vi "Station_1_Detection.vi"() -> ()   [LabVIEW 2011]
uses:
  <vilib>/userDefined/High Color/IMAQdx.ctl
  <vilib>/Utility/file.llb/Write To Spreadsheet File (string).vi
  <vilib>/vision/driver/NI_Vision_Acquisition_Software.lvlib
  <vilib>/vision/NI_Vision_Development_Module.lvlib
panel:
  in  "Minimum Match Score":sgl=900.0
  in  "Text File Information":path=path "C:/Users/Kevin/Documents/Masters (Semester 2)/MEng Thesis/LabVIEW_CompleteV3/TextFiles"
  in  "Saved Image Location":path=path "C:/Users/Kevin/Documents/Masters (Semester 2)/MEng Thesis/LabVIEW_CompleteV3/ImagesFiles"
  in  "Template Location":path=path "C:/Users/Kevin/Documents/Masters (Semester 2)/MEng Thesis/LabVIEW_CompleteV3/Templates/Shape"
  in  "Colour Selection":enum32{"Default", "Automatic", "Manual"}(radio)
  out "Created Colours":u32[](array[colorbox])
  out "Switch Ready":bool
  out "Colours Ready":bool
  in  "Run Search":bool
  out "Running":bool
  out "Results Cluster":T2 {"Colour Code" format="%.0x"}
  out "Image File":string
  in  "Selected Colours":u32[](array[colorbox])
  in  "Full Program Stop":bool
  out "Image Out":T1(plugin-control)
  out "Results Information":string[][](table)
  out "No Shapes Found":bool
  out "Shape(s) Found":bool
  out "Image Iteration":u32
  out "Saving":bool
  out "Image Name":string
  # "Kevin Mulkearn\n11124725\nUniversity of Limerick"
  # "Instructions:\n1. Select File Locations.\n2. Run application.\n3. Generate/Select Colours.\n4. Select 'START' button."
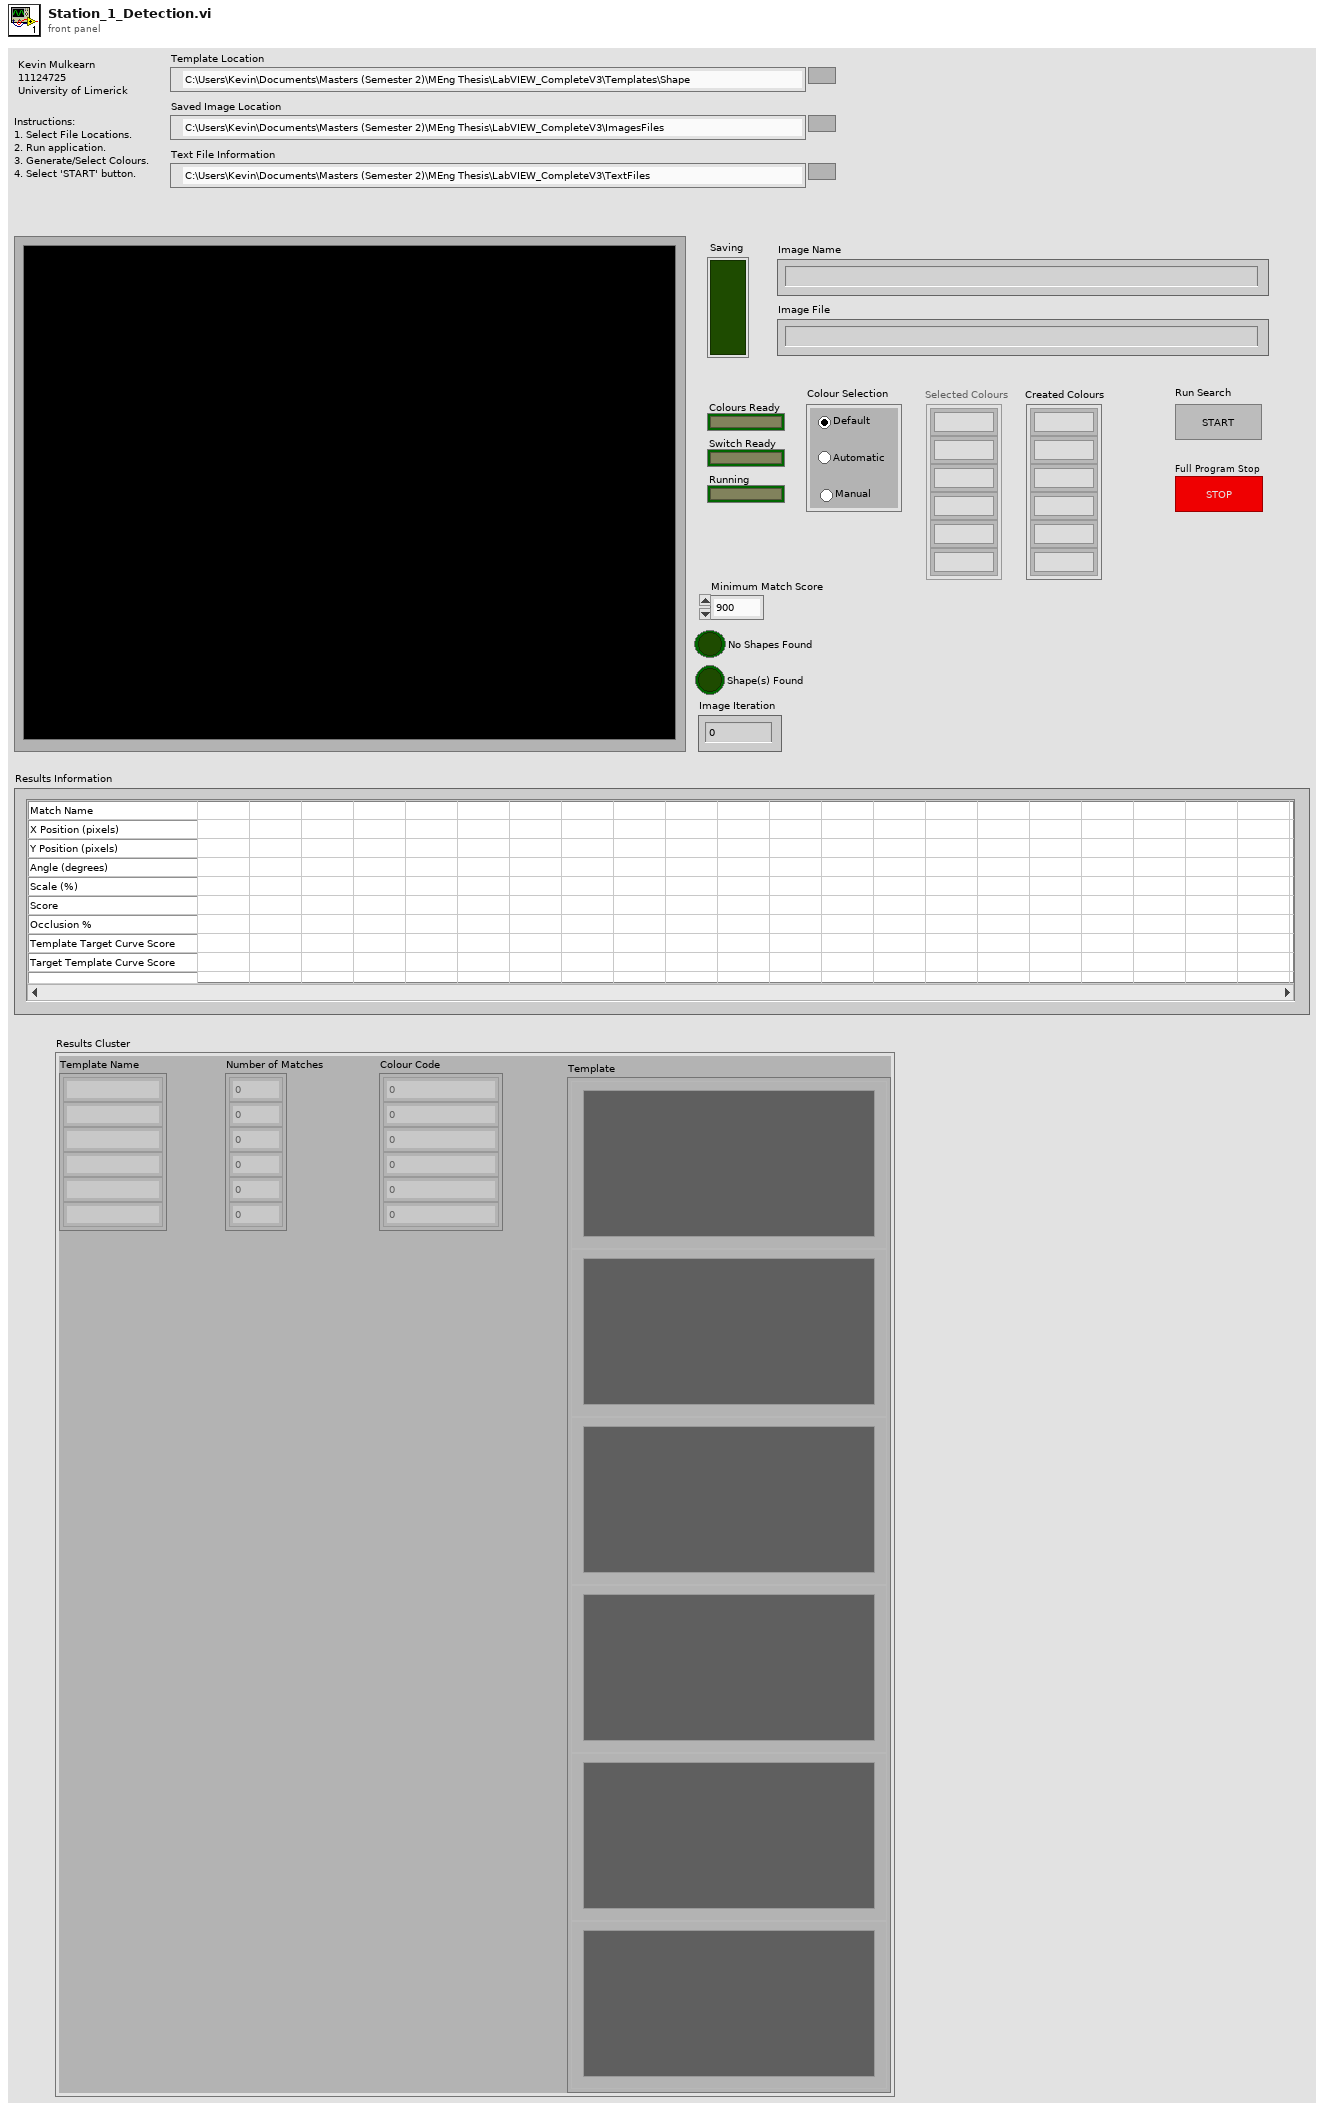
[diagram p1: front panel]
types:
  T1 = typedef "IMAQ Image.ctl" = refnum<image>
  T2 = cluster{"Number of Matches":i32[], "Colour Code":u32[], "Template":T1[], "Template Name":string[]}
  T3 = typedef "IMAQdx.ctl" = refnum<k21>
  T4 = cluster{"Rotation":bool, "Scale":bool, "Occlusion":bool, "Reserved":bool, "Reserved":bool, "Reserved":bool}
  T5 = cluster{"Match Geometric Pattern Setup Data":string, "Number of Matches":i32, "Minimum Match Score":sgl}
  T6 = typedef "IMAQ GM Multiple Template.ctl" = refnum<k20>
  T7 = enum8{"Enabled", "Disabled", "Disabled and Grayed Out"}
  T8 = typedef "IMAQ GM Match Report.ctl" = cluster{"Position":cluster{"x":sgl, "y":sgl}, "Angle":sgl, "Scale":sgl, "Score":sgl, "Bounding Box":cluster{"x":sgl, "y":sgl}[], "Contrast Reversed":bool, "Occlusion %":sgl, "Template Target Curve Score":sgl, "Target Template Curve Score":sgl, "Correlation Score":sgl}
  T9 = cluster{"Number of Matches":i32[], u32[], T1[], string[]}
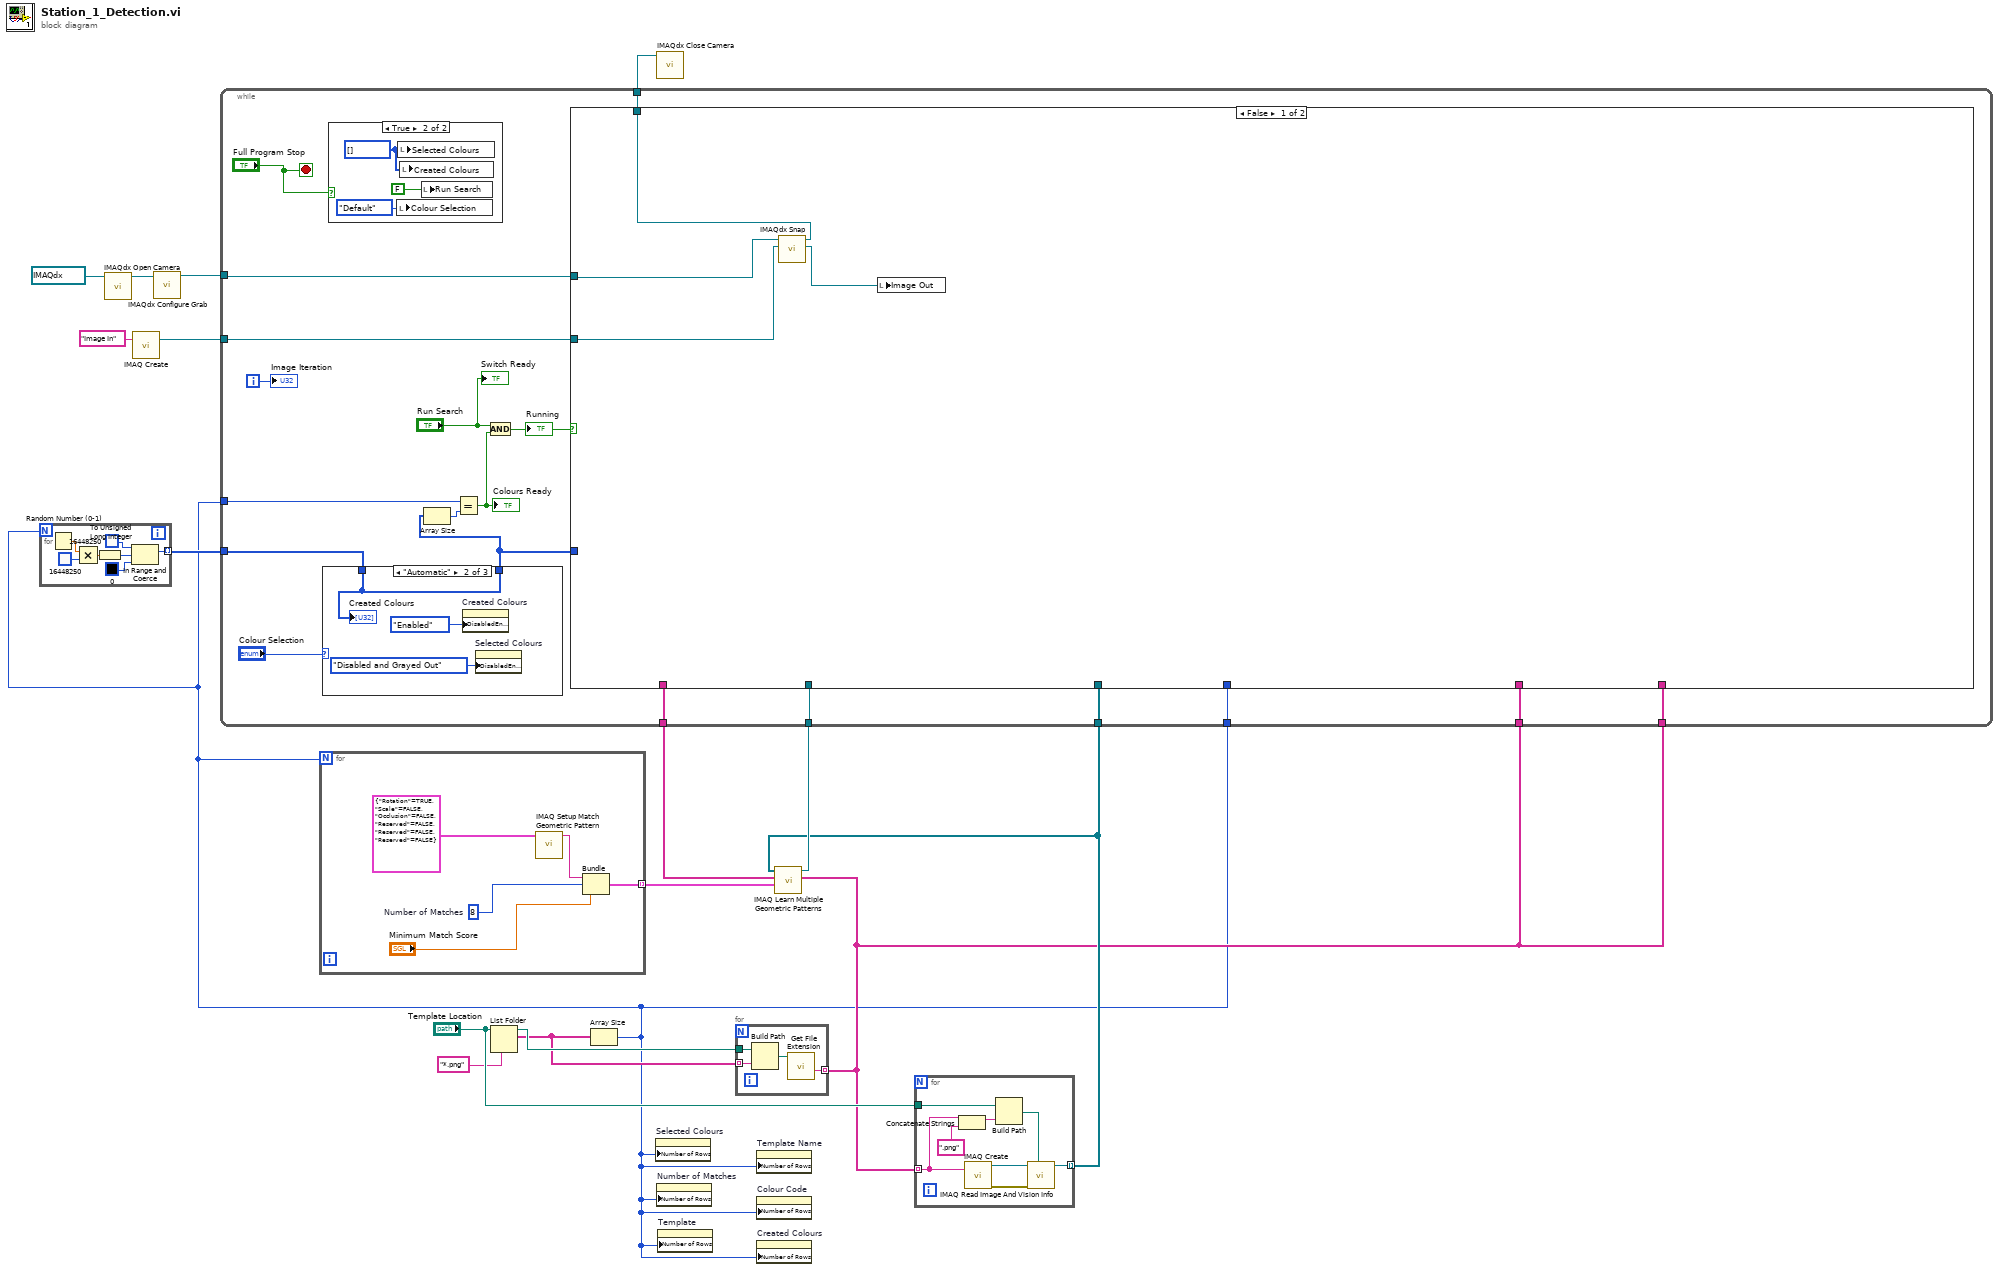
[diagram p0: block diagram]
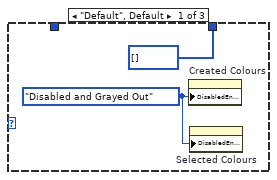
[diagram p2: hidden frame]
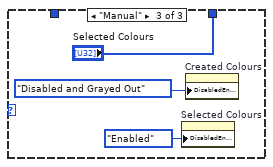
[diagram p3: hidden frame]
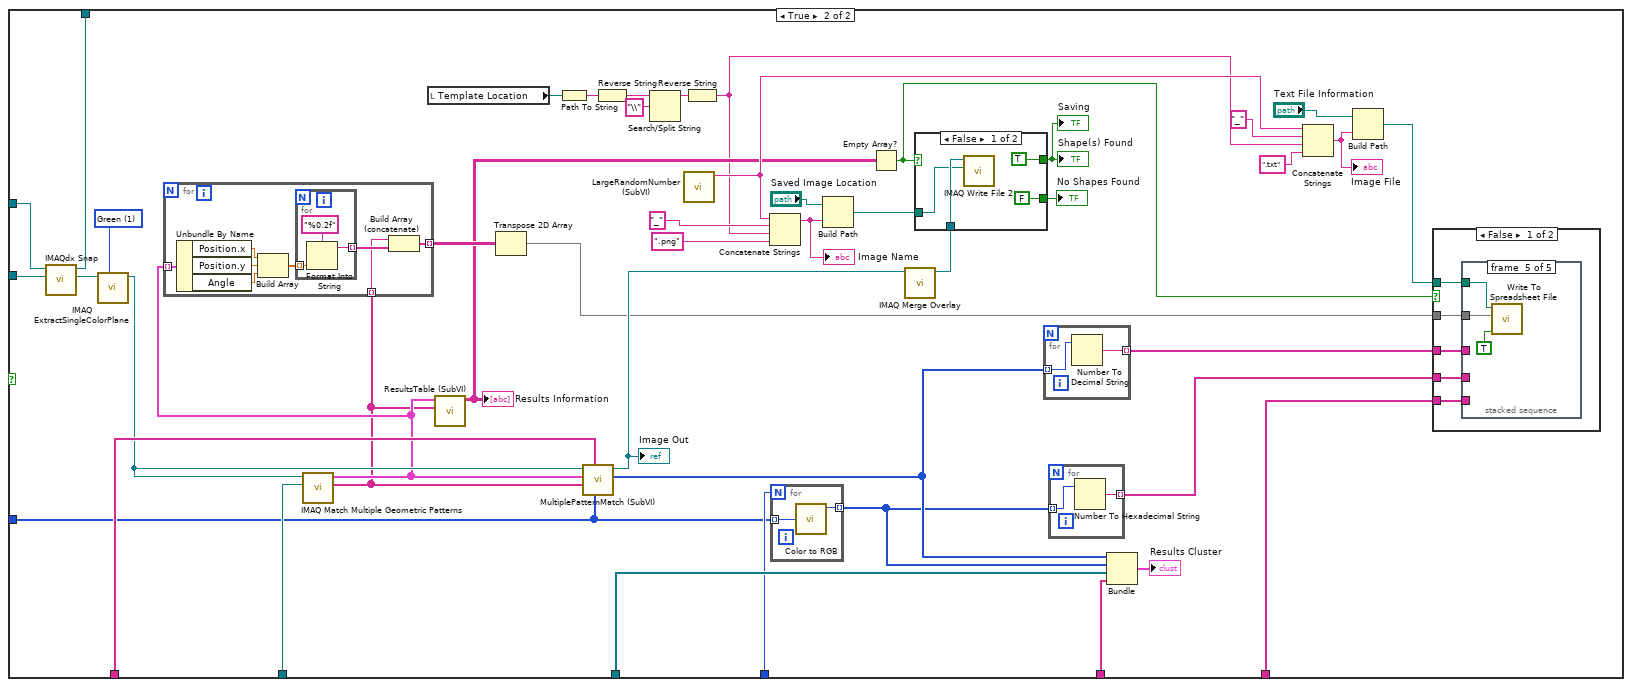
[diagram p5: hidden frame]
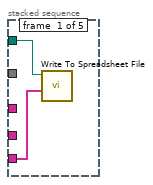
[diagram p6: hidden frame]
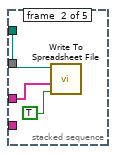
[diagram p7: hidden frame]
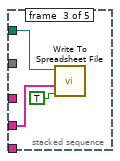
[diagram p8: hidden frame]
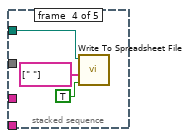
[diagram p9: hidden frame]
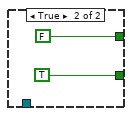
[diagram p11: hidden frame]
diagram:
  n1 = call <vilib>:"IMAQdx Open Camera.vi"("Session In"=T3 "cam2") -> ("Session Out"=w15:T3)  [unwired: 9 in, 1 out]
  n2 = call "IMAQ Create"("Image Name"="Image In") -> ("New Image"=w11:T1)  [unwired: 4 in, 1 out]
  n3 = call <vilib>:"IMAQdx Configure Grab.vi"("Session In"=w15) -> ("Session Out"=w14:T3)  [unwired: 9 in, 1 out]
  n4 = List Folder(path="Template Location", pattern="*.png") -> (path out=w6:path, filenames=w5:string[])  [unwired: 2 in, 2 out]
  n5 = Array Size(array=w5) -> (size(s)=w1:i32)
  n6 = for {
    N: w1 -> [_]
    tunnel: [w17] -> w2 mode=indexing
    n7 = Random Number (0-1)() -> (number: 0 to 1=w18:dbl)
    n8 = Multiply(x=w18, y=u32 16448250 ("Lightest Limit 2")) -> (x*y=w22:dbl)
    n9 = To Unsigned Long Integer(number=w22) -> (unsigned 32bit integer=w23:u32)
    n10 = In Range and Coerce(upper limit=u32 16448250 ("Lightest Limit"), x=w23, lower limit=u32 0 ("Darkest Limit")) -> (coerced(x)=w17:u32)  [unwired: 1 out]
  }
  n11 = for {
    N: w1 -> [_]
    tunnel: [w26] -> w10 mode=indexing
    w25 = 8  # Number of Matches
    n12 = call "IMAQ Setup Match Geometric Pattern"("Match Mode"=T4 {"Rotation"=TRUE, "Scale"=FALSE, "Occlusion"=FALSE, "Reserved"=FALSE, "Reserved"=FALSE, "Reserved"=FALSE}) -> ("Match Geometric Pattern Setup Data"=w27:string)  [unwired: 9 in, 1 out]
    n13 = Bundle("Match Geometric Pattern Setup Data"=w27, "Number of Matches"=w25, "Minimum Match Score"="Minimum Match Score") -> (w26:T5)  [unwired: 1 in]
  }
  n14 = property on="Selected Colours" class="Arr (strict)"("Number of Rows"=w1) -> ()  [unwired: 2 in, 2 out]
  n15 = property on="Number of Matches" class="Arr (strict)"("Number of Rows"=w1) -> ()  [unwired: 2 in, 2 out]
  n16 = property on="Template" class="Arr (strict)"("Number of Rows"=w1) -> ()  [unwired: 2 in, 2 out]
  n17 = for {
    tunnel: w6 -> [w32]
    tunnel: w5 -> [w31] mode=indexing
    tunnel: [w29] -> w3 mode=indexing
    n18 = Build Path(base path=w32, name or relative path=w31) -> (appended path=w30:path)
    n19 = call <vilib>:"Get File Extension.vi"("file"=w30) -> ("filename without extension"=w29:string)  [unwired: 7 in, 3 out]
  }
  n20 = property on="Template Name" class="Arr (strict)"("Number of Rows"=w1) -> ()  [unwired: 2 in, 2 out]
  n21 = property on="Colour Code" class="Arr (strict)"("Number of Rows"=w1) -> ()  [unwired: 2 in, 2 out]
  n22 = property on="Created Colours" class="Arr (strict)"("Number of Rows"=w1) -> ()  [unwired: 2 in, 2 out]
  n23 = for {
    tunnel: w3 -> [w38] mode=indexing
    tunnel: [w39] -> w7 mode=indexing
    tunnel: "Template Location" -> [w34]
    n24 = Concatenate Strings(w38, ".png" ("string")) -> (w37:string)
    n25 = call "IMAQ Create"("Image Name"=w38) -> ("New Image"=w40:T1, "error out"=w35:errorcluster)  [unwired: 3 in, 1 out]
    n26 = Build Path(base path=w34, name or relative path=w37) -> (appended path=w33:path)
    n27 = call "IMAQ Read Image And Vision Info"("File Path"=w33, "error in (no error)"=w35, "Image"=w40) -> ("Image Out"=w39:T1)  [unwired: 1 in, 7 out]
  }
  n28 = call "IMAQ Learn Multiple Geometric Patterns"("Default Match Options"=w10, "Template Labels"=w3, "Template Images"=w7) -> ("Multiple Template (out)"=w9:T6)  [unwired: 7 in, 1 out]
  n29 = while {
    tunnel: w14 -> [w59]
    tunnel: [w57] -> w13
    tunnel: w11 -> [w58]
    tunnel: w9 -> [w56]
    tunnel: w3 -> [w54]
    tunnel: w7 -> [w53]
    tunnel: w3 -> [w51]
    tunnel: w3 -> [w52]
    tunnel: w1 -> [w50]
    tunnel: w1 -> [w45]
    tunnel: w2 -> [w42]
    i -> [w55]
    stop <- "Full Program Stop" stop-if-true
    n30 = case shown="\"Automatic\"" "Colour Selection" {
      tunnel: [u32[] [] ("Select Colours") w64 "Selected Colours"] -> w43
      tunnel: w42 -> [_ w64 _]
      frame "Default", Default {
        w60 = T7."Disabled and Grayed Out" ("Disabled")
        n31 = property on="Created Colours" class="Arr (strict)"("DisabledEnum"=w60) -> ()  [unwired: 2 in, 2 out]
        n32 = property on="Selected Colours" class="Arr (strict)"("DisabledEnum"=w60) -> ()  [unwired: 2 in, 2 out]
      }
      frame "Automatic" {
        n33 = property on="Created Colours" class="Arr (strict)"("DisabledEnum"=T7."Enabled" ("Disabled")) -> ()  [unwired: 2 in, 2 out]
        n34 = property on="Selected Colours" class="Arr (strict)"("DisabledEnum"=T7."Disabled and Grayed Out" ("Disabled")) -> ()  [unwired: 2 in, 2 out]
        "Created Colours" <- w64
      }
      frame "Manual" {
        n35 = property on="Selected Colours" class="Arr (strict)"("DisabledEnum"=T7."Enabled" ("Disabled")) -> ()  [unwired: 2 in, 2 out]
        n36 = property on="Created Colours" class="Arr (strict)"("DisabledEnum"=T7."Disabled and Grayed Out" ("Disabled")) -> ()  [unwired: 2 in, 2 out]
      }
    }
    n37 = case shown="True" "Full Program Stop" {
      frame False {
      }
      frame True {
        w68 = u32[] []
        n38 = local write "Colour Selection"(enum32{"Default", "Automatic", "Manual"}."Default" ("Colour Selection Method")) -> ()
        n39 = local write "Selected Colours"(w68) -> ()
        n40 = local write "Created Colours"(w68) -> ()
        n41 = local write "Run Search"(FALSE ("Boolean")) -> ()
      }
    }
    n42 = Array Size(array=w43) -> (size(s)=w46:i32)
    n43 = Equal?(x=w45, y=w46) -> (x = y?=w47:bool)
    "Colours Ready" <- w47
    n44 = And(x="Run Search", y=w47) -> (x .and. y?=w49:bool)
    "Running" <- w49
    n45 = case shown="False" w49 {
      tunnel: w59 -> [w74 w119]
      tunnel: w58 -> [w73 w118]
      tunnel: [w71 w117] -> w57
      tunnel: w56 -> [_ w114]
      tunnel: w54 -> [_ w107]
      tunnel: w53 -> [_ w104]
      tunnel: w52 -> [_ w94]
      tunnel: w51 -> [_ w87]
      tunnel: w50 -> [_ w86]
      tunnel: w43 -> [_ w85]
      frame False {
        n46 = call <vilib>:"IMAQdx Snap.vi"("Image In"=w73, "Session In"=w74) -> ("Image Out"=w72:T1, "Session Out"=w71:T3)  [unwired: 7 in, 1 out]
        n47 = local write "Image Out"(w72) -> ()
      }
      frame True {
        w116 = 1 items=["Red", "Green", "Blue", "Hue", "Saturation", "Luminance", "Value", "Intensity"] ("Color Plane")
        n48 = call <vilib>:"IMAQdx Snap.vi"("Image In"=w118, "Session In"=w119) -> ("Image Out"=w115:T1, "Session Out"=w117:T3)  [unwired: 7 in, 1 out]
        n49 = call "IMAQ ExtractSingleColorPlane"("Color Plane"=w116, "Image Src"=w115) -> ("Image Dst Out"=w105:T1)  [unwired: 8 in, 1 out]
        n50 = call "IMAQ Match Multiple Geometric Patterns"("Multiple Template"=w114, "Image"=w105) -> ("Matched Labels"=w84:string[], "Matches (pixel)"=w92:T8[])  [unwired: 6 in, 2 out]
        n51 = for {
          tunnel: w92 -> [w127] mode=indexing
          tunnel: [w121] -> w90 mode=indexing
          tunnel: w84 -> [w120] mode=indexing
          n52 = Unbundle By Name(w127) -> ("Position.x"=w125:sgl, "Position.y"=w126:sgl, "Angle"=w124:sgl)
          n53 = Build Array(w125, w126, w124) -> (w123:sgl[])
          n54 = for {
            tunnel: w123 -> [w130] mode=indexing
            tunnel: [w128] -> w122 mode=indexing
            n55 = Format Into String(format string="%0.2f", w130) -> (resulting string=w128:string)  [unwired: 2 in, 1 out]
          }
          n56 = Build Array (concatenate)(w120, w122) -> (w121:string[])
        }
        n57 = local read "Template Location"() -> (w75:path)
        n58 = call "ResultsTable (SubVI).vi"("Match Labels"=w84, "Matches"=w92) -> ("Text Results"=w89:string[][])  [unwired: 8 in, 1 out]
        "Results Information" <- w89
        n59 = Transpose 2D Array(2D array=w90) -> (transposed array=w88:string[][])
        n60 = Path To String(path=w75) -> (string=w81:string)
        n61 = call "MultiplePatternMatch (SubVI).vi"("Label Colors"=w85, "Learned Labels"=w107, "Match Labels"=w84, "Match Results"=w92, "Refnum in"=w105) -> ("Number of Matches"=w98:i32[], "Refnum out"=w106:T1)  [unwired: 4 in, 1 out]
        "Image Out" <- w106
        n62 = Reverse String(1:w81) -> (0:w82:string)
        n63 = Search/Split String(string=w82, search string/char (-)="\\") -> (substring before match=w83:string)  [unwired: 1 in, 2 out]
        n64 = call "LargeRandomNumber (SubVI).vi"() -> ("Random Number"=w91:string)  [unwired: 11 in]
        n65 = Reverse String(1:w83) -> (0:w76:string)
        n66 = Concatenate Strings(w91, "_", w76, ".png") -> (w108:string)
        "Image Name" <- w108
        n67 = for {
          N: w86 -> [_]
          tunnel: w85 -> [w155] mode=indexing
          tunnel: [w154] -> w97 mode=indexing
          n68 = call <vilib>:"Color to RGB.vi"("Color"=w155) -> ("Resolved Color"=w154:u32)  [unwired: 3 out]
        }
        n69 = Build Path(base path="Saved Image Location", name or relative path=w108) -> (appended path=w111:path)
        n70 = Empty Array?(array=w89) -> (empty?=w103:bool)
        n71 = call "IMAQ Merge Overlay"("Image Src"=w106) -> ("Image Dst Out"=w110:T1)  [unwired: 4 in, 6 out]
        n72 = case shown="False" w103 {
          tunnel: [TRUE FALSE] -> w109
          tunnel: [FALSE TRUE] -> w113
          tunnel: w110 -> [w157 _]
          tunnel: w111 -> [w156 _]
          frame False {
            n73 = call-poly "IMAQ Write File 2"("File Path"=w156, "Image"=w157) -> ()  [unwired: 8 in, 2 out]
          }
          frame True {
          }
        }
        "No Shapes Found" <- w113
        "Shape(s) Found" <- w109
        "Saving" <- w109
        n74 = for {
          tunnel: w98 -> [w134] mode=indexing
          tunnel: [w133] -> w96 mode=indexing
          n75 = Number To Decimal String(number=w134) -> (decimal integer string=w133:string)  [unwired: 1 in]
        }
        n76 = for {
          tunnel: w97 -> [w132] mode=indexing
          tunnel: [w131] -> w95 mode=indexing
          n77 = Number To Hexadecimal String(2:w132) -> (0:w131:string)  [unwired: 1 in]
        }
        n78 = Bundle("Number of Matches"=w98, w97, w104, w94) -> (→"Results Cluster":T9)  [unwired: 1 in]
        n79 = Concatenate Strings(w91, "_", w76, ".txt") -> (w100:string)
        "Image File" <- w100
        n80 = Build Path(base path="Text File Information", name or relative path=w100) -> (appended path=w99:path)
        n81 = case shown="False" w103 {
          tunnel: w99 -> [w136 _]
          tunnel: w87 -> [w139 _]
          tunnel: w96 -> [w138 _]
          tunnel: w95 -> [w137 _]
          tunnel: w88 -> [w135 _]
          frame False {
            n82 = stacked-sequence {
              tunnel: w139 -> [w141 _ _ _ _]
              tunnel: w138 -> [_ w144 _ _ _]
              tunnel: w137 -> [_ _ w146 _ _]
              tunnel: w136 -> [w140 w142 w145 w149 w152]
              tunnel: w135 -> [_ _ _ _ w151]
              frame #0 {
                n83 = call-poly <vilib>:"Write To Spreadsheet File.vi"("1D data"=w141, "file path (dialog if empty)"=w140) -> ()  [unwired: 6 in, 1 out]
              }
              frame #1 {
                n84 = call-poly <vilib>:"Write To Spreadsheet File.vi"("append to file? (new file:F)"=TRUE, "1D data"=w144, "file path (dialog if empty)"=w142) -> ()  [unwired: 5 in, 1 out]
              }
              frame #2 {
                n85 = call-poly <vilib>:"Write To Spreadsheet File.vi"("append to file? (new file:F)"=TRUE, "1D data"=w146, "file path (dialog if empty)"=w145) -> ()  [unwired: 5 in, 1 out]
              }
              frame #3 {
                n86 = call-poly <vilib>:"Write To Spreadsheet File.vi"("append to file? (new file:F)"=TRUE, "1D data"=string[] [" "], "file path (dialog if empty)"=w149) -> ()  [unwired: 5 in, 1 out]
              }
              frame #4 {
                n87 = call-poly <vilib>:"Write To Spreadsheet File.vi"("append to file? (new file:F)"=TRUE, "2D data"=w151, "file path (dialog if empty)"=w152) -> ()  [unwired: 5 in, 1 out]
              }
            }
          }
          frame True {
          }
        }
      }
    }
    "Image Iteration" <- w55
    "Switch Ready" <- "Run Search"
  }
  n88 = call <vilib>:"IMAQdx Close Camera.vi"("Session In"=w13) -> ()  [unwired: 10 in, 1 out]
